vi "FRCts20_WebMethods_Convert_Events_PUT.vi"(8 "error in (no error)":errorcluster, 11 "Single Event in":T3) -> (0 "error out":errorcluster, 3 "Event In":T1)   [LabVIEW 2014, in "FRCts20_WebMethods.lvlib"]
uses:
  FRCts20_WebMethods.lvlib
  Backend/source/VI Source/FRCts20_Backend_API/FRCts20_Backend_API_Event.ctl
  Backend/source/VI Source/FRCts20_Backend_API/FRCts20_Backend_API_SW.ctl
  Web Method Public Interface/FRCts20_WebMethods_ctl_teamIdentifier.ctl
  Web Method Public Interface/FRCts20_WebMethods_ctl_singleEvent.ctl
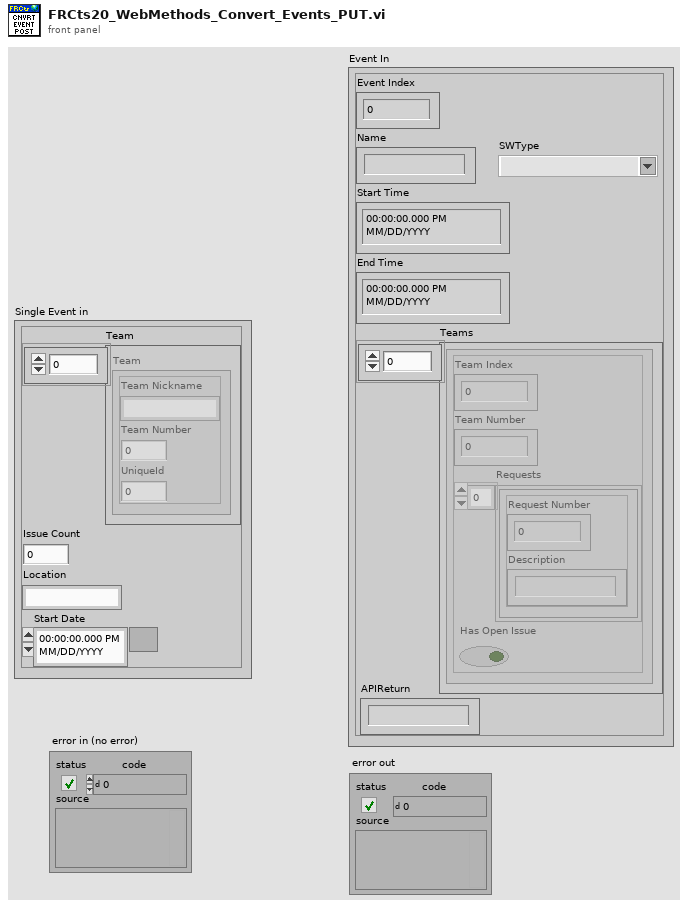
[diagram p1: front panel]
types:
  T1 = typedef "FRCts20_Backend_API.lvlib/FRCts20_Backend_API_Event.ctl" = cluster{"Event Index":u32, "Name":string, "Start Time":timestamp, "End Time":timestamp, "Teams":cluster{"Team Index":u32, "Team Number":u32, "Requests":cluster{"Request Number":u32, "Description":string}[], "Has Open Issue":bool}[], "SWType":T2, "APIReturn":string}
  T2 = typedef "FRCts20_Backend_API.lvlib/FRCts20_Backend_API_SW.ctl" = string
  T3 = typedef "FRCts20_WebMethods.lvlib/FRCts20_WebMethods_ctl_singleEvent.ctl" = cluster{"Team":T4[], "Issue Count":i32, "Location":string, "Start Date ":timestamp}
  T4 = typedef "FRCts20_WebMethods.lvlib/FRCts20_WebMethods_ctl_teamIdentifier.ctl" = cluster{"Team Nickname":string, "Team Number ":u32, "UniqueId":u32}
  T5 = cluster{"Team Index":u32, "Team Number":u32, "Requests":cluster{"Request Number":u32, "Description":string}[], "Has Open Issue":bool}[]
  T6 = cluster{"Team Index":u32, "Team Number":u32, "Requests":cluster{"Request Number":u32, "Description":string}[], "Has Open Issue":bool}
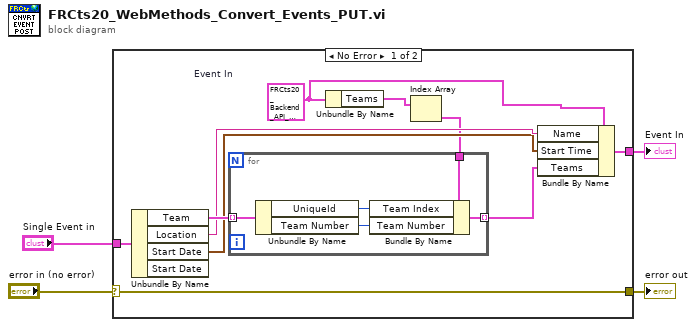
[diagram p0: block diagram]
diagram:
  n1 = case shown="No Error" "error in (no error)" {
    selector: "error in (no error)" -> [w12 w20]
    tunnel: [w12 w20] -> w3
    tunnel: "Single Event in" -> [w14 _]
    tunnel: [w13 _] -> w1
    frame No Error {
      w5 = T1 {"Event Index"=0, "Name"="", "Start Time"=timestamp(0 s since 1904-01-01), "End Time"=timestamp(0 s since 1904-01-01), "Teams"=[], "SWType"="", "APIReturn"=""}  # Event In
      n2 = Unbundle By Name(w14) -> ("Team"=w11:T4[], "Location"=w9:string, "Start Date"=w8:timestamp)  [unwired: 1 out]
      n3 = Unbundle By Name(w5) -> ("Teams"=w7:T5)
      n4 = Index Array(array=w7) -> (element=w6:T6)  [unwired: 1 in]
      n5 = for {
        tunnel: w11 -> [w19] mode=indexing
        tunnel: [w16] -> w10 mode=indexing
        tunnel: w6 -> [w15]
        n6 = Unbundle By Name(w19) -> ("UniqueId"=w18:u32, "Team Number"=w17:u32)
        n7 = Bundle By Name(cluster=w15, "Team Index"=w18, "Team Number"=w17) -> (w16:T6)
      }
      n8 = Bundle By Name(cluster=w5, "Name"=w9, "Start Time"=w8, "Teams"=w10) -> (w13:T1)
    }
    frame Error {
    }
  }
  "Event In" <- w1
  "error out" <- w3
